vi "kalman_filter.vi"(11 "u":dbl, 12 "Q":dbl=1.0, 14 "R":dbl=0.1) -> (4 "xest":dbl)   [LabVIEW 2014]
panel:
  # "more aggressive means\nsmaller R (measurement noise covariance)\nbigger Q (process noise covariance)"
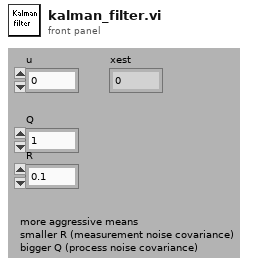
[diagram p1: front panel]
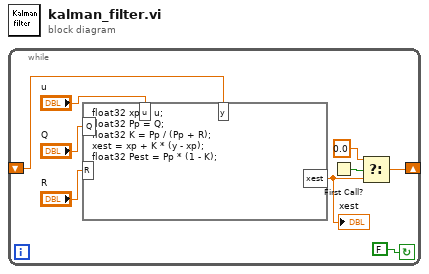
[diagram p0: block diagram]
diagram:
  n1 = while {
    shift-right: [w1] -> _
    shift-left: _ -> [w5]
    stop <- FALSE continue-if-true
    n2 = formula code="float32 xp = u;\nfloat32 Pp = Q;\nfloat32 K = Pp / (Pp + R);\nxest = xp + K * (y - xp);\nfloat32 Pest = Pp * (1 - K);"("Q"="Q", "u"="u", "R"="R", "y"=w5) -> ("xest"=w2:dbl)
    "xest" <- w2
    n3 = First Call?() -> (First Call?: T/F=w4:bool)
    n4 = Select(t=0.0, s=w4, f=w2) -> (s? t:f=w1:dbl)
  }
